vi "test - NESTED read with submodule.vi"(8 "error in (no error)":errorcluster, 11 "TestCase in":refnum<class "csm-ini-variable-addon.lvclass">) -> (0 "error out":errorcluster, 3 "TestCase out":refnum<class "csm-ini-variable-addon.lvclass">)   [LabVIEW 2017, in "csm-ini-variable-addon.lvclass"]
uses:
  csm-ini-variable-addon.lvclass
  INI-Static-Variable-Support/INI-Static-Variable-Support.lvlib
panel:
  # "Connector Pane"
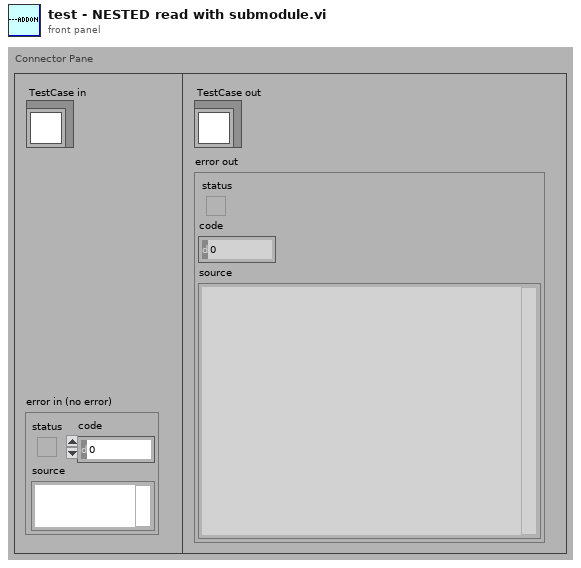
[diagram p1: front panel]
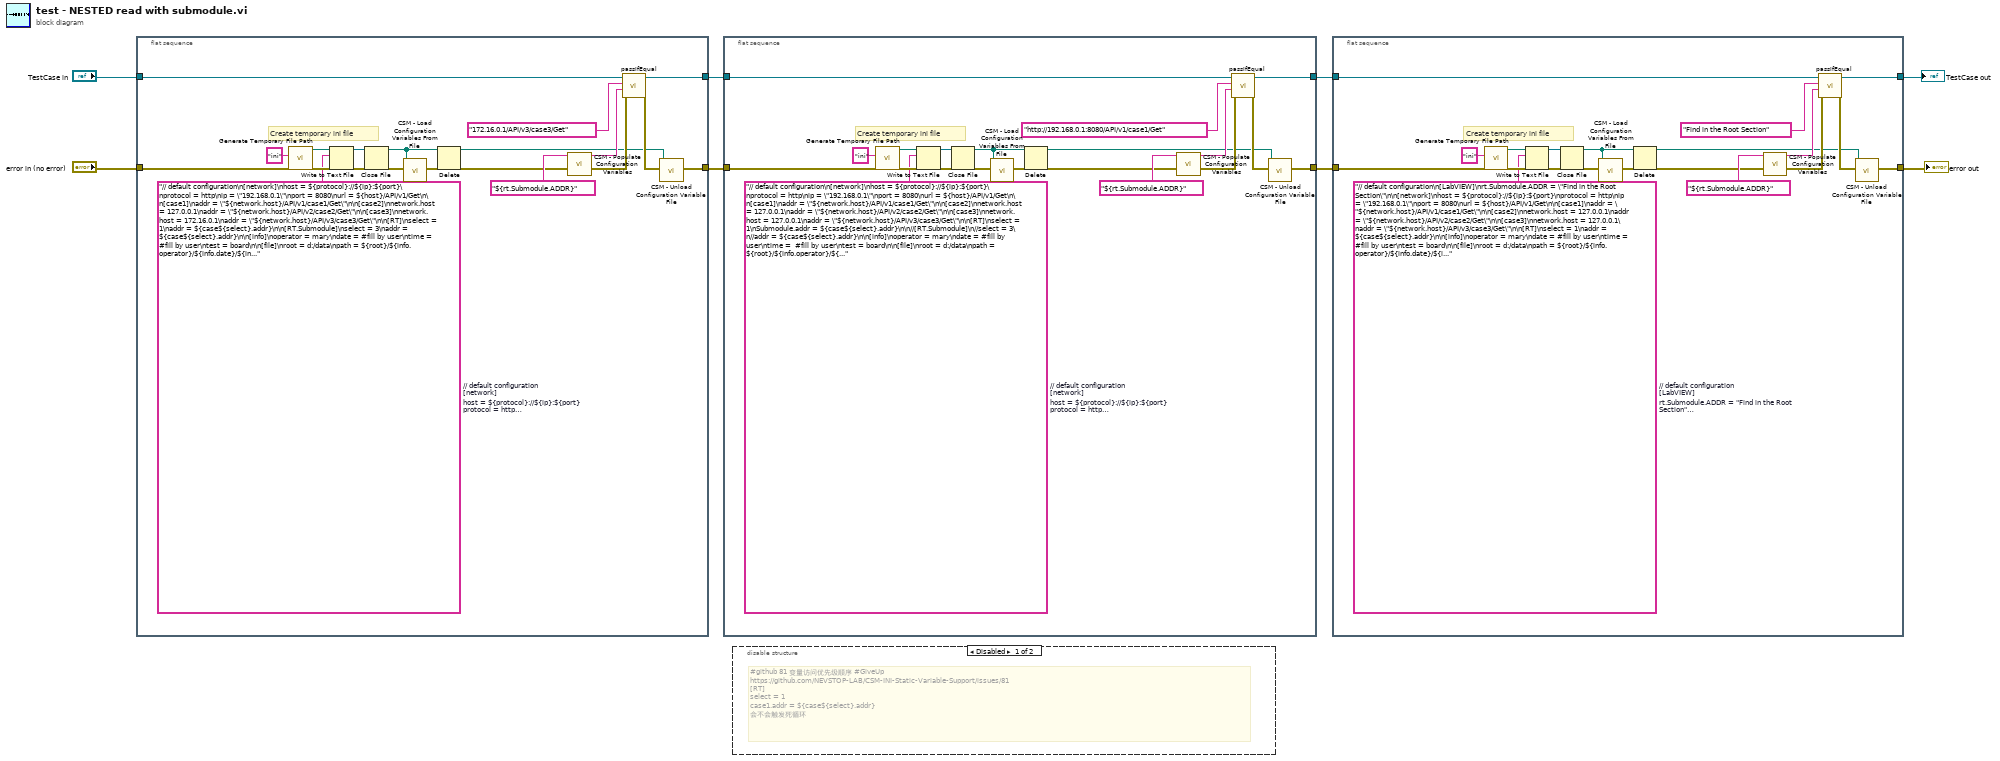
[diagram p0: block diagram]
diagram:
  n1 = flat-sequence {
    tunnel: "error in (no error)" -> [w28]
    tunnel: [w13] -> w6
    tunnel: "TestCase in" -> [w12]
    tunnel: [w9] -> w5
    frame #0 {
      w21 = "// default configuration\n[network]\nhost = ${protocol}://${ip}:${port}\nprotocol = http\nip = \"192.168.0.1\"\nport = 8080\nurl = ${host}/API/v1/Get\n\n[case1]\naddr = \"${network.host}/API/v1/case1/Get\"\n\n[case2]\nnetwork.host = 127.0.0.1\naddr = \"${network.host}/API/v2/case2/Get\"\n\n[case3]\nnetwork.host = 172.16.0.1\naddr = \"${network.host}/API/v3/case3/Get\"\n\n[RT]\nselect = 1\naddr = ${case${select}.addr}\n\n[RT.Submodule]\nselect = 3\naddr = ${case${select}.addr}\n\n[info]\noperator = mary\ndate = #fill by user\ntime =  #fill by user\ntest = board\n\n[file]\nroot = d:/data\npath = ${root}/${info.operator}/${info.date}/${info.test}${info.time}.tdms"  # // default configuration [network] host = ${protocol}://${ip}:${port} protocol = http ip = "192.168.0.1" port = 8080 url = ${host}/API/v1/Get  [case1] addr = "${network.host}/API/v1/case1/Get"  [case2] network.host = 127.0.0.1 addr = "${network.host}/API/v2/case2/Get"  [case3] network.host = 172.16.0.1 addr = "${network.host}/API/v3/case3/Get"  [RT] select = 1 addr = ${case${select}.addr}  [RT.Submodule] select = 3 addr = ${case${select}.addr}  [info] operator = mary date = #fill by user time =  #fill by user test = board  [file] root = d:/data path = ${root}/${info.operator}/${info.date}/${info.test}${info.time}.tdms
      # "Create temporary ini file"
      n2 = call <vilib>:"Generate Temporary File Path.vi"("error in (no error)"=w28, "Temporary File Extension (tmp)"="ini") -> ("error out"=w27:errorcluster, "Unique Temporary File Path"=w24:path)  [unwired: 8 in]
      n3 = Write to Text File(file (use dialog)=w24, text=w21, error in=w27) -> (refnum out=w23:refnum<file>, error out=w25:errorcluster)  [unwired: 1 in, 1 out]
      n4 = Close File(refnum=w23, error in=w25) -> (path=w19:path, error out=w22:errorcluster)
      n5 = call "CSM - Load Configuration Variables From File.vi"("error in (no error)"=w22, "Path"=w19) -> ("error out"=w20:errorcluster)  [unwired: 7 in]
      n6 = Delete(path (use dialog)=w19, error in=w20) -> (deleted path=w10:path, error out=w14:errorcluster)  [unwired: 3 in, 1 out]
      n7 = call "CSM - Populate Configuration Variables.vi"("error in (no error)"=w14, "String in"="${rt.Submodule.ADDR}") -> ("error out"=w17:errorcluster, "String out"=w18:string)  [unwired: 6 in]
      n8 = call-dynamic "passIfEqual.vi"("error in (no error)"=w17, "y"=w18, "x"="172.16.0.1/API/v3/case3/Get" ("${rt.addr}"), "TestCase in"=w12) -> ("error out"=w11:errorcluster, "TestCase out"=w13:refnum<class "csm-ini-variable-addon.lvclass">)  [unwired: 6 in]
      n9 = call "CSM - Unload Configuration Variable File.vi"("error in (no error)"=w11, "Path"=w10) -> ("error out"=w9:errorcluster)  [unwired: 7 in]
    }
  }
  n10 = flat-sequence {
    tunnel: w5 -> [w48]
    tunnel: [w33] -> w4
    tunnel: w6 -> [w32]
    tunnel: [w29] -> w3
    frame #0 {
      w41 = "// default configuration\n[network]\nhost = ${protocol}://${ip}:${port}\nprotocol = http\nip = \"192.168.0.1\"\nport = 8080\nurl = ${host}/API/v1/Get\n\n[case1]\naddr = \"${network.host}/API/v1/case1/Get\"\n\n[case2]\nnetwork.host = 127.0.0.1\naddr = \"${network.host}/API/v2/case2/Get\"\n\n[case3]\nnetwork.host = 127.0.0.1\naddr = \"${network.host}/API/v3/case3/Get\"\n\n[RT]\nselect = 1\nSubmodule.addr = ${case${select}.addr}\n\n//[RT.Submodule]\n//select = 3\n//addr = ${case${select}.addr}\n\n[info]\noperator = mary\ndate = #fill by user\ntime =  #fill by user\ntest = board\n\n[file]\nroot = d:/data\npath = ${root}/${info.operator}/${info.date}/${info.test}${info.time}.tdms"  # // default configuration [network] host = ${protocol}://${ip}:${port} protocol = http ip = "192.168.0.1" port = 8080 url = ${host}/API/v1/Get  [case1] addr = "${network.host}/API/v1/case1/Get"  [case2] network.host = 127.0.0.1 addr = "${network.host}/API/v2/case2/Get"  [case3] network.host = 127.0.0.1 addr = "${network.host}/API/v3/case3/Get"  [RT] select = 1 Submodule.addr = ${case${select}.addr}  //[RT.Submodule] //select = 3 //addr = ${case${select}.addr}  [info] operator = mary date = #fill by user time =  #fill by user test = board  [file] root = d:/data path = ${root}/${info.operator}/${info.date}/${info.test}${info.time}.tdms
      # "Create temporary ini file"
      n11 = call <vilib>:"Generate Temporary File Path.vi"("error in (no error)"=w48, "Temporary File Extension (tmp)"="ini") -> ("error out"=w47:errorcluster, "Unique Temporary File Path"=w44:path)  [unwired: 8 in]
      n12 = Write to Text File(file (use dialog)=w44, text=w41, error in=w47) -> (refnum out=w43:refnum<file>, error out=w45:errorcluster)  [unwired: 1 in, 1 out]
      n13 = Close File(refnum=w43, error in=w45) -> (path=w39:path, error out=w42:errorcluster)
      n14 = call "CSM - Load Configuration Variables From File.vi"("error in (no error)"=w42, "Path"=w39) -> ("error out"=w40:errorcluster)  [unwired: 7 in]
      n15 = Delete(path (use dialog)=w39, error in=w40) -> (deleted path=w30:path, error out=w34:errorcluster)  [unwired: 3 in, 1 out]
      n16 = call "CSM - Populate Configuration Variables.vi"("error in (no error)"=w34, "String in"="${rt.Submodule.ADDR}") -> ("error out"=w37:errorcluster, "String out"=w38:string)  [unwired: 6 in]
      n17 = call-dynamic "passIfEqual.vi"("error in (no error)"=w37, "y"=w38, "x"="http://192.168.0.1:8080/API/v1/case1/Get" ("${rt.addr}"), "TestCase in"=w32) -> ("error out"=w31:errorcluster, "TestCase out"=w33:refnum<class "csm-ini-variable-addon.lvclass">)  [unwired: 6 in]
      n18 = call "CSM - Unload Configuration Variable File.vi"("error in (no error)"=w31, "Path"=w30) -> ("error out"=w29:errorcluster)  [unwired: 7 in]
    }
  }
  n19 = disable-structure shown="Disabled" {
    frame Disabled {
      # "#github 81 变量访问优先级顺序 #GiveUp\nhttps://github.com/NEVSTOP-LAB/CSM-INI-Static-Variable-Support/issues/81\n[RT]\nselect = 1\ncase1.addr = ${case${select}.addr}\n会不会触发死循环"
    }
    frame Enabled {
    }
  }
  n20 = flat-sequence {
    tunnel: w3 -> [w68]
    tunnel: [w53] -> w2
    tunnel: w4 -> [w52]
    tunnel: [w49] -> w1
    frame #0 {
      w61 = "// default configuration\n[LabVIEW]\nrt.Submodule.ADDR = \"Find in the Root Section\"\n\n[network]\nhost = ${protocol}://${ip}:${port}\nprotocol = http\nip = \"192.168.0.1\"\nport = 8080\nurl = ${host}/API/v1/Get\n\n[case1]\naddr = \"${network.host}/API/v1/case1/Get\"\n\n[case2]\nnetwork.host = 127.0.0.1\naddr = \"${network.host}/API/v2/case2/Get\"\n\n[case3]\nnetwork.host = 127.0.0.1\naddr = \"${network.host}/API/v3/case3/Get\"\n\n[RT]\nselect = 1\naddr = ${case${select}.addr}\n\n[info]\noperator = mary\ndate = #fill by user\ntime =  #fill by user\ntest = board\n\n[file]\nroot = d:/data\npath = ${root}/${info.operator}/${info.date}/${info.test}${info.time}.tdms"  # // default configuration [LabVIEW] rt.Submodule.ADDR = "Find in the Root Section"  [network] host = ${protocol}://${ip}:${port} protocol = http ip = "192.168.0.1" port = 8080 url = ${host}/API/v1/Get  [case1] addr = "${network.host}/API/v1/case1/Get"  [case2] network.host = 127.0.0.1 addr = "${network.host}/API/v2/case2/Get"  [case3] network.host = 127.0.0.1 addr = "${network.host}/API/v3/case3/Get"  [RT] select = 1 addr = ${case${select}.addr}  [info] operator = mary date = #fill by user time =  #fill by user test = board  [file] root = d:/data path = ${root}/${info.operator}/${info.date}/${info.test}${info.time}.tdms
      # "Create temporary ini file"
      n21 = call <vilib>:"Generate Temporary File Path.vi"("error in (no error)"=w68, "Temporary File Extension (tmp)"="ini") -> ("error out"=w67:errorcluster, "Unique Temporary File Path"=w64:path)  [unwired: 8 in]
      n22 = Write to Text File(file (use dialog)=w64, text=w61, error in=w67) -> (refnum out=w63:refnum<file>, error out=w65:errorcluster)  [unwired: 1 in, 1 out]
      n23 = Close File(refnum=w63, error in=w65) -> (path=w59:path, error out=w62:errorcluster)
      n24 = call "CSM - Load Configuration Variables From File.vi"("error in (no error)"=w62, "Path"=w59) -> ("error out"=w60:errorcluster)  [unwired: 7 in]
      n25 = Delete(path (use dialog)=w59, error in=w60) -> (deleted path=w50:path, error out=w54:errorcluster)  [unwired: 3 in, 1 out]
      n26 = call "CSM - Populate Configuration Variables.vi"("error in (no error)"=w54, "String in"="${rt.Submodule.ADDR}") -> ("error out"=w57:errorcluster, "String out"=w58:string)  [unwired: 6 in]
      n27 = call-dynamic "passIfEqual.vi"("error in (no error)"=w57, "y"=w58, "x"="Find in the Root Section" ("${rt.addr}"), "TestCase in"=w52) -> ("error out"=w51:errorcluster, "TestCase out"=w53:refnum<class "csm-ini-variable-addon.lvclass">)  [unwired: 6 in]
      n28 = call "CSM - Unload Configuration Variable File.vi"("error in (no error)"=w51, "Path"=w50) -> ("error out"=w49:errorcluster)  [unwired: 7 in]
    }
  }
  "error out" <- w1
  "TestCase out" <- w2
